vi "MecaWheel_GetAll.vi"(11 "MECA_WHEEL_SPEEDS":T1 {"RearRightSpeed" format="%19.3f"; "RearLeftSpeed" format="%19.3f"; "FrontRightSpeed" format="%19.3f"; "FrontLeftSpeed" format="%19.3f"}) -> (0 "RearRightSpeed":dbl format="%19.3f", 1 "RearLeftSpeed":dbl format="%19.3f", 2 "FrontRightSpeed":dbl format="%19.3f", 3 "FrontLeftSpeed":dbl format="%19.3f")   [LabVIEW 2019, in "Trajectory_Library.lvlib"]
doc: "Returns the individual wheel speeds from a MecanumDriveWheelSpeeds data structure.\n\nParameters:\n - Meca_wheel_speeds - Data structure\n\nReturns:\n - Left Front Speed - Speed of left front wheel (meters/sec)\n - Right Front Speed - Speed of right front wheel (meters/sec)\n - Left Rear Speed - Speed of left rear wheel (meters/sec)\n - Right Rear Speed - Speed of right rear wheel (meters/sec)"
uses:
  Trajectory_Library.lvlib
  TypeDef/MECA_WHEEL_SPEEDS.ctl
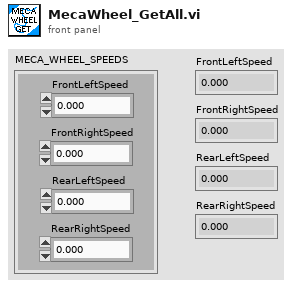
[diagram p1: front panel]
types:
  T1 = typedef "Trajectory_Library.lvlib/MECA_WHEEL_SPEEDS.ctl" = cluster{"FrontLeftSpeed":dbl, "FrontRightSpeed":dbl, "RearLeftSpeed":dbl, "RearRightSpeed":dbl}
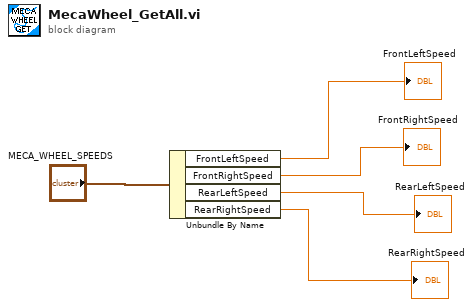
[diagram p0: block diagram]
diagram:
  n1 = Unbundle By Name("MECA_WHEEL_SPEEDS") -> ("FrontLeftSpeed"=→"FrontLeftSpeed":dbl, "FrontRightSpeed"=→"FrontRightSpeed":dbl, "RearLeftSpeed"=→"RearLeftSpeed":dbl, "RearRightSpeed"=→"RearRightSpeed":dbl)
